vi "Iterative Read.vi"(5 "Username":string, 6 "Password":string, 7 "Address":string, 8 "Error In":errorcluster) -> (0 "Error Out":errorcluster)   [LabVIEW 2018, in "Tests.lvlib" / "SFTP File.lvlib"]
uses:
  SFTP File.lvlib
  <vilib>/addons/_JKI Toolkits/Caraya/classes/Test/Test.lvclass
  <vilib>/addons/_JKI Toolkits/Caraya/classes/Assert/Assert.lvclass
  src/Toolkit/API/SFTP File/SFTP File.lvclass
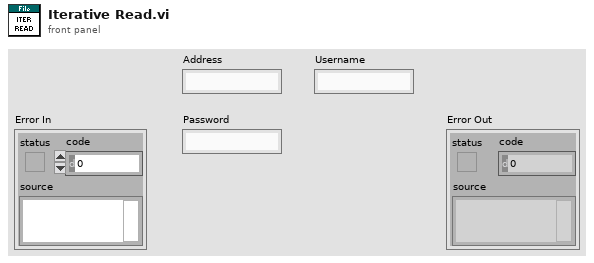
[diagram p1: front panel]
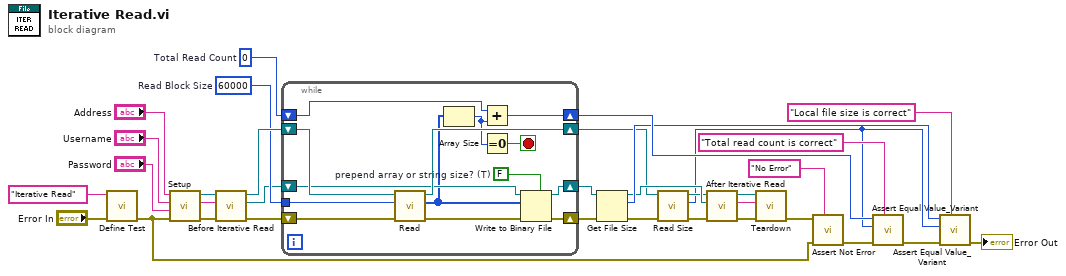
[diagram p0: block diagram]
diagram:
  w9 = 60000  # Read Block Size
  w18 = 0  # Total Read Count
  n1 = call <vilib>:"Define Test.vi"("error in (no error)"="Error In", "Label (VI Title)"="Iterative Read") -> ("error out"=w28:errorcluster)  [unwired: 9 in]
  n2 = call "Setup.vi"("Error In"=w28, "Password"="Password", "Username"="Username", "Address"="Address") -> ("Error Out"=w20:errorcluster, "Temporary File"=w19:string, "SFTP"=w21:refnum<class "SFTP.lvclass">)  [unwired: 5 in]
  n3 = call "Before Iterative Read.vi"("Error In"=w20, "Temporary File"=w19, "SFTP"=w21) -> ("Error Out"=w8:errorcluster, "Local File"=w7:refnum<file>, "SFTP File"=w25:refnum<class "SFTP File.lvclass">)  [unwired: 6 in]
  n4 = while {
    shift-right: [w44] -> w4
    shift-left: w25 -> [w46]
    shift-right: [w40] -> w16
    shift-left: w8 -> [w45]
    shift-right: [w41] -> w17
    shift-left: w7 -> [w42]
    shift-right: [w47] -> w15
    shift-left: w18 -> [w48]
    tunnel: w9 -> [w36]
    stop <- w37 stop-if-true
    w39 = FALSE  # prepend array or string size? (T)
    n5 = call "Read.vi"("Error In"=w45, "Max Data Length"=w36, "SFTP File In"=w46) -> ("Error Out"=w43:errorcluster, "Data"=w38:u8[], "SFTP File Out"=w44:refnum<class "SFTP File.lvclass">)  [unwired: 6 in]
    n6 = Array Size(array=w38) -> (size(s)=w35:i32)
    n7 = Add(x=w48, y=w35) -> (x+y=w47:i32)
    n8 = Equal To 0?(x=w35) -> (x = 0?=w37:bool)
    n9 = Write to Binary File(file (use dialog)=w42, data=w38, error in=w43, 5:w39) -> (refnum out=w41:refnum<file>, error out=w40:errorcluster)  [unwired: 2 in, 1 out]
  }
  n10 = Get File Size(file=w17, error in=w16) -> (refnum out=w6:refnum<file>, size (in bytes)=w11:i64, 0:w5:errorcluster)
  n11 = call "Read Size.vi"("Error In"=w5, "SFTP File In"=w4) -> ("Error Out"=w3:errorcluster, "File Size"=w1:u64, "SFTP File Out"=w2:refnum<class "SFTP File.lvclass">)  [unwired: 7 in]
  n12 = call "After Iterative Read.vi"("Error In"=w3, "Local File"=w6, "SFTP File"=w2) -> ("Error Out"=w23:errorcluster, "Remote Path"=w22:string, "SFTP"=w24:refnum<class "SFTP.lvclass">)  [unwired: 6 in]
  n13 = call "Teardown.vi"("Error In"=w23, "Temporary File"=w22, "SFTP"=w24) -> ("Error Out"=w27:errorcluster)  [unwired: 8 in]
  n14 = call <vilib>:"Assert Not Error.vi"("Label"="No Error", "error in (no error)"=w28, "Not Error?"=w27) -> ("error out"=w26:errorcluster)  [unwired: 8 in]
  n15 = call <vilib>:"Assert Equal Value_Variant.vi"("Label"="Total read count is correct", "error in (no error)"=w26, "Y"=w1, "X"=w15) -> ("error out"=w13:errorcluster)  [unwired: 7 in]
  n16 = call <vilib>:"Assert Equal Value_Variant.vi"("Label"="Local file size is correct", "error in (no error)"=w13, "Y"=w1, "X"=w11) -> ("error out"=→"Error Out":errorcluster)  [unwired: 7 in]
